vi "Test Create Complex Number.vi"() -> ()   [LabVIEW 2014]
uses:
  Complex Numbers.lvlib
panel:
  out "Complex":i32
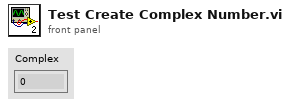
[diagram p1: front panel]
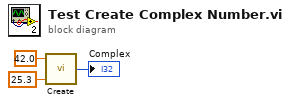
[diagram p0: block diagram]
diagram:
  n1 = call "Create.vi"("Imag"=25.3, "Real"=42.0) -> ("Complex"=→"Complex":u32)  [unwired: 3 in]
